vi "DictionaryLearnings.vi"   [LabVIEW 2020]
doc: "Polymorphic VI for dictionary learning models"
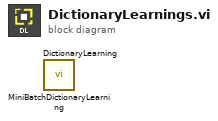
[diagram p0: block diagram]
diagram:
  n1 = call "MiniBatchDictionaryLearning.vi"() -> ()  [unwired: 10 in, 2 out]
  n2 = call "DictionaryLearning.vi"() -> ()  [unwired: 10 in, 2 out]
